vi "Log Data DBL.vi"(8 "error in":errorcluster, 9 "Time Stamp":timestamp format="%<%x %.3X>T", 10 "Data":dbl, 11 "Action Point in":refnum<class "Action Point.lvclass">) -> (0 "error out":errorcluster, 3 "Action Point out":refnum<class "Action Point.lvclass">)   [LabVIEW 2024, in "Action Point.lvclass"]
uses:
  Action Point.lvclass
  Action Point.lvclass/Action Point.ctl
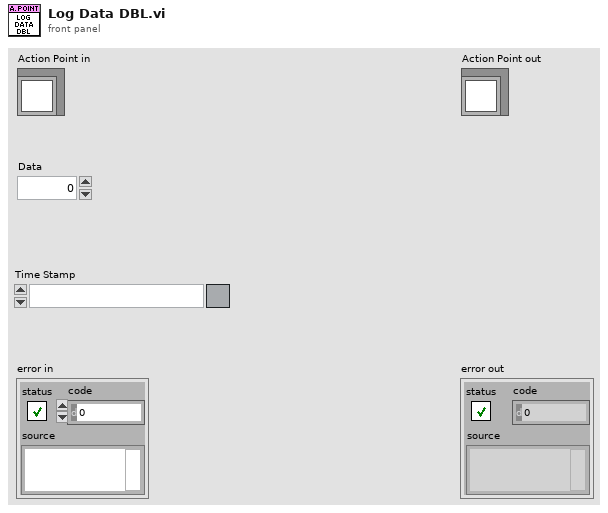
[diagram p1: front panel]
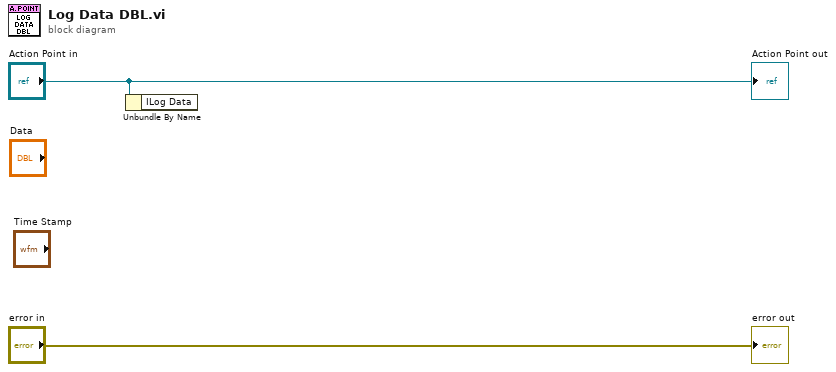
[diagram p0: block diagram]
diagram:
  n1 = Unbundle By Name("Action Point in") -> ()  [unwired: 1 out]
  "error out" <- "error in"
  "Action Point out" <- "Action Point in"
